vi "count_electrons.vi"(7 "Raw Image Data In":T2) -> (8 "Raw Image Data Out":T2, 13 "Electron Counts Out":i32)   [LabVIEW 2023]
uses:
  <vilib>/vision/Image Controls.llb/IMAQ Image.ctl
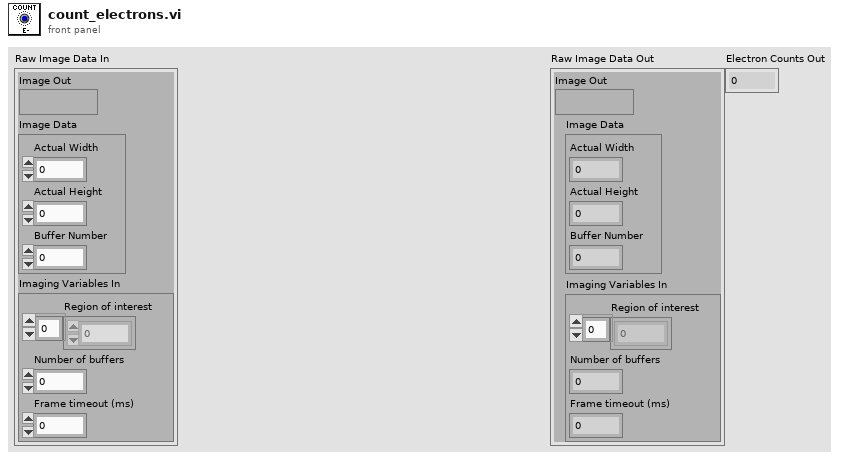
[diagram p1: front panel]
types:
  T1 = typedef "IMAQ Image.ctl" = refnum<image>
  T2 = cluster{"Image Out":T1, "Image Data":cluster{"Actual Width":u32, "Actual Height":u32, "Buffer Number":i32}, "Imaging Variables In":cluster{"Region of interest":i32[], "Number of buffers":u32, "Frame timeout (ms)":u32}}
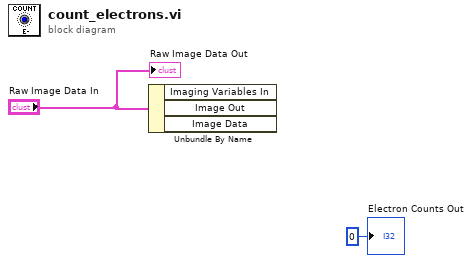
[diagram p0: block diagram]
diagram:
  n1 = Unbundle By Name("Raw Image Data In") -> ()  [unwired: 3 out]
  "Raw Image Data Out" <- "Raw Image Data In"
  "Electron Counts Out" <- 0
